vi "Pos_iniciales3.vi"() -> ()   [LabVIEW 2020]
panel:
  in  "Pos_Iniciales3":T1
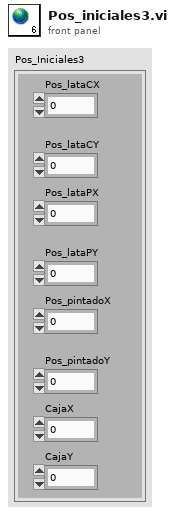
[diagram p1: front panel]
types:
  T1 = cluster{"Pos_lataCX":dbl, "Pos_lataCY":dbl, "Pos_lataPX":dbl, "Pos_lataPY":dbl, "Pos_pintadoX":dbl, "Pos_pintadoY":dbl, "CajaX":dbl, "CajaY":dbl}
diagram:
